vi "gen MB frame -Delayed ON Relay.vi"(9 "Half Period(sec)":dbl, 10 "Relays IDs":T1=3 items=["Relay 1"=3, "Relay 2"=8, "Relay 3"=13, "Relay 4"=18, "Relay 5"=23, "Relay 6"=28, "Relay 7"=33, "Relay 8"=38], 11 "Dev Addr":u8=1 format="%x") -> (3 "MB frame":string)   [LabVIEW 2016, in "MB _relays.lvlib"]
uses:
  MB _relays.lvlib
  type defs/Relays IDs flash.ctl
panel:
  out "*(type *) &x":string
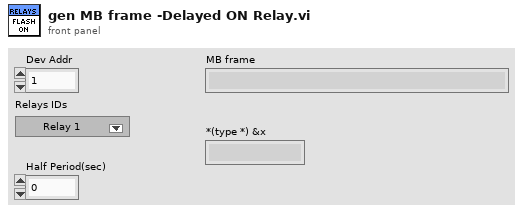
[diagram p1: front panel]
types:
  T1 = typedef "MB _relays.lvlib/Relays IDs flash.ctl" = u16
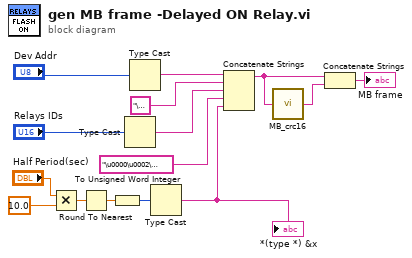
[diagram p0: block diagram]
diagram:
  n1 = Multiply(x="Half Period(sec)", y=10.0) -> (x*y=w7:dbl)
  n2 = Round To Nearest(number=w7) -> (nearest integer value=w6:dbl)
  n3 = To Unsigned Word Integer(number=w6) -> (unsigned 16bit integer=w3:u16)
  n4 = Type Cast(x="Relays IDs") -> (*(type *) &x=w5:string)  [unwired: 1 in]
  n5 = Type Cast(x="Dev Addr") -> (*(type *) &x=w14:string)  [unwired: 1 in]
  n6 = Type Cast(x=w3) -> (*(type *) &x=w2:string)  [unwired: 1 in]
  "*(type *) &x" <- w2
  n7 = Concatenate Strings(w14, "\u0010", w5, "\u0000\u0002\u0004\u0000\u0004", w2) -> (w12:string)
  n8 = call "MB_crc16.vi"("message"=w12) -> ("CRC16"=w11:string)  [unwired: 4 in]
  n9 = Concatenate Strings(w12, w11) -> (→"MB frame":string)
